vi "Untitled 1.vi"() -> ()   [LabVIEW 2013]
uses:
  lightfield-automation-labview/VIs/ClientServerMode/CS_LFAClassGlobal.vi
  lightfield-automation-labview/LightField Automation.lvclass
panel:
  in  "Grating Index (0 -> n-1)":i32
  out "Center Wavelenght":dbl
  in  "Center Wavelength":dbl
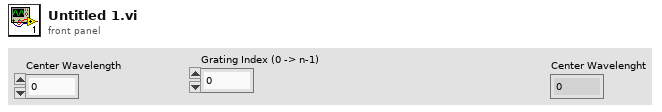
[diagram p1: front panel]
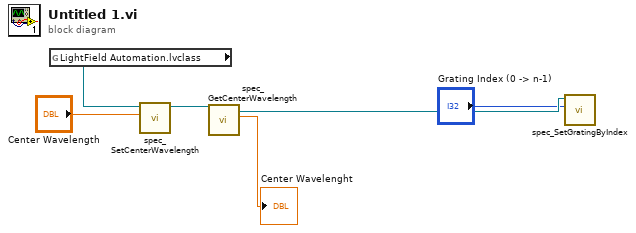
[diagram p0: block diagram]
diagram:
  n1 = global read "CS_LFAClassGlobal.vi" "LightField Automation.lvclass"() -> (w5:refnum<class "LightField Automation.lvclass">)
  n2 = call "spec_SetCenterWavelength.vi"("Center Wavelength"="Center Wavelength", "LightField Automation in"=w5) -> ("LightField Automation out"=w6:refnum<class "LightField Automation.lvclass">)  [unwired: 8 in, 1 out]
  n3 = call "spec_GetCenterWavelength.vi"("LightField Automation in"=w6) -> ("Center Wavelenght"=→"Center Wavelenght":dbl, "LightField Automation out"=w2:refnum<class "LightField Automation.lvclass">)  [unwired: 8 in, 1 out]
  n4 = call "spec_SetGratingByIndex.vi"("Grating Index (0 -> n-1)"="Grating Index (0 -> n-1)", "LightField Automation in"=w2) -> ()  [unwired: 8 in, 2 out]
